vi "CheckX.vi"(9 "BoolText.Text":string, 10 "BoolText.Text 2":string, 11 "BoolText.Text 3":string) -> (3 "Boolean":bool)   [LabVIEW 2018]
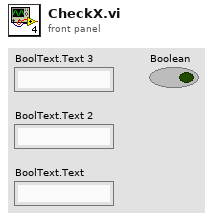
[diagram p1: front panel]
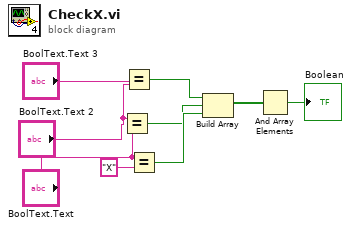
[diagram p0: block diagram]
diagram:
  n1 = Equal?(x="BoolText.Text 2", y="BoolText.Text") -> (x = y?=w6:bool)
  n2 = Equal?(x="BoolText.Text 3", y="BoolText.Text 2") -> (x = y?=w5:bool)
  n3 = Equal?(x="BoolText.Text", y="X") -> (x = y?=w7:bool)
  n4 = Build Array(w5, w6, w7) -> (w8:bool[])
  n5 = And Array Elements(Boolean array=w8) -> (logical AND=→"Boolean":bool)
